vi "mbdmaboot_Host_nodownload.vi"() -> ()   [LabVIEW 2015]
uses:
  <vilib>/FPGAPlugInAG/USRP X310; 294xR; 295xR/niLvFpga_Open_USRP X310; 294xR; 295xR.vi
  <vilib>/rvi/interface/common/dynamic/niFpgaDynamicAddResources.vi
  <vilib>/FPGAPlugInAG/Dynamic/niLvFpga_Download_Dynamic.vi
  <vilib>/FPGAPlugInAG/Dynamic/niLvFpga_Run_Dynamic.vi
  <vilib>/Utility/error.llb/Error Cluster From Error Code.vi
  <vilib>/rvi/errors/niLvFpgaAdjustHostInterfaceError.vi
  <vilib>/FPGAPlugInAG/Dynamic/niLvFpga_Close_Dynamic.vi
  <vilib>/rvi/interface/nirviOpenFPGA/nirviOpenFPGA.xnode
  FPGA Bitfiles/mb-dmaboot_FPGATarget_mbdmaboottopLeve_XKhxGc+VYWY.lvbitx
  <vilib>/rvi/interface/nirviMethod/nirviMethod.xnode
  <vilib>/rvi/interface/nirviReadWriteControl/nirviReadWriteControl.xnode
  <vilib>/rvi/interface/nirviCloseFPGA/nirviCloseFPGA.xnode
  <vilib>/FPGAPlugInAG/Dynamic/niLvFpga_ReadFifo_Dynamic.vi
  <vilib>/rvi/errors/niLvFpgaMergeErrorWithErrorCode.vi
  NiFpgaLv.dll
  <vilib>/rvi/interface/Simulation/niFpgaSimulationCallBeginRW.vi
panel:
  in  "ub1\\reset_rtl":bool
  out "Console out (readonly) 2":string
  out "C":u32
  in  "B":u32
  in  "A":u32
  in  "stop":bool
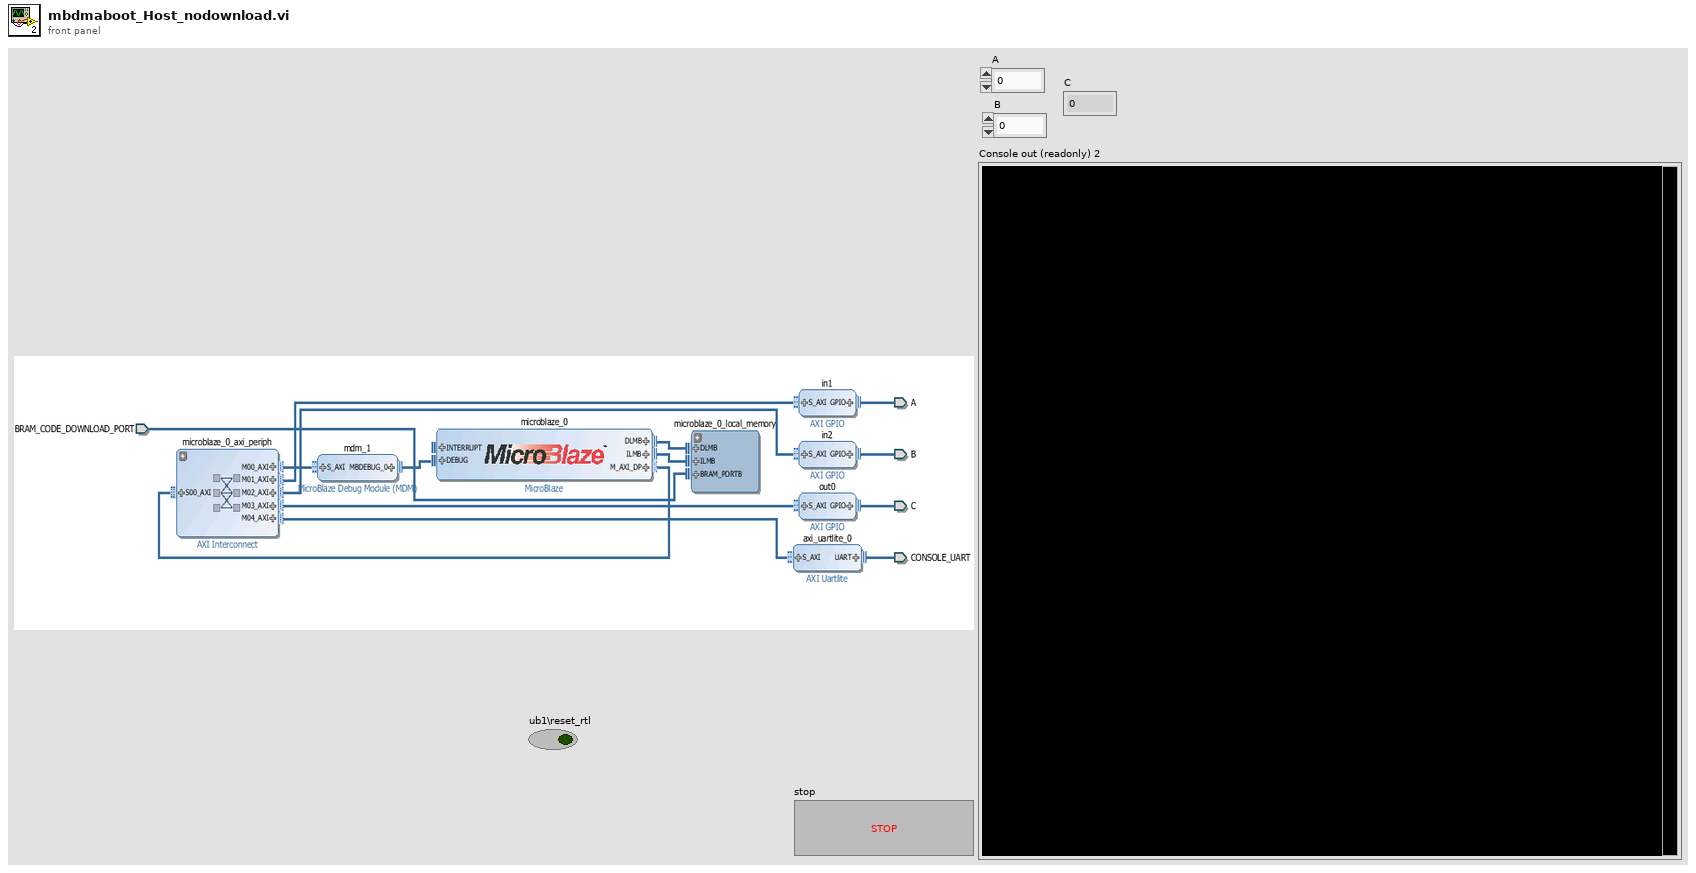
[diagram p1: front panel]
types:
  T1 = cluster{"Baud (ticks)":u32, "CharacterSize":u8, "Parity":enum8{"None", "Even", "Odd"}, "Stop Bits":enum8{"1.0", "1.5", "2.0"}, "Spacing (ticks)":u32}
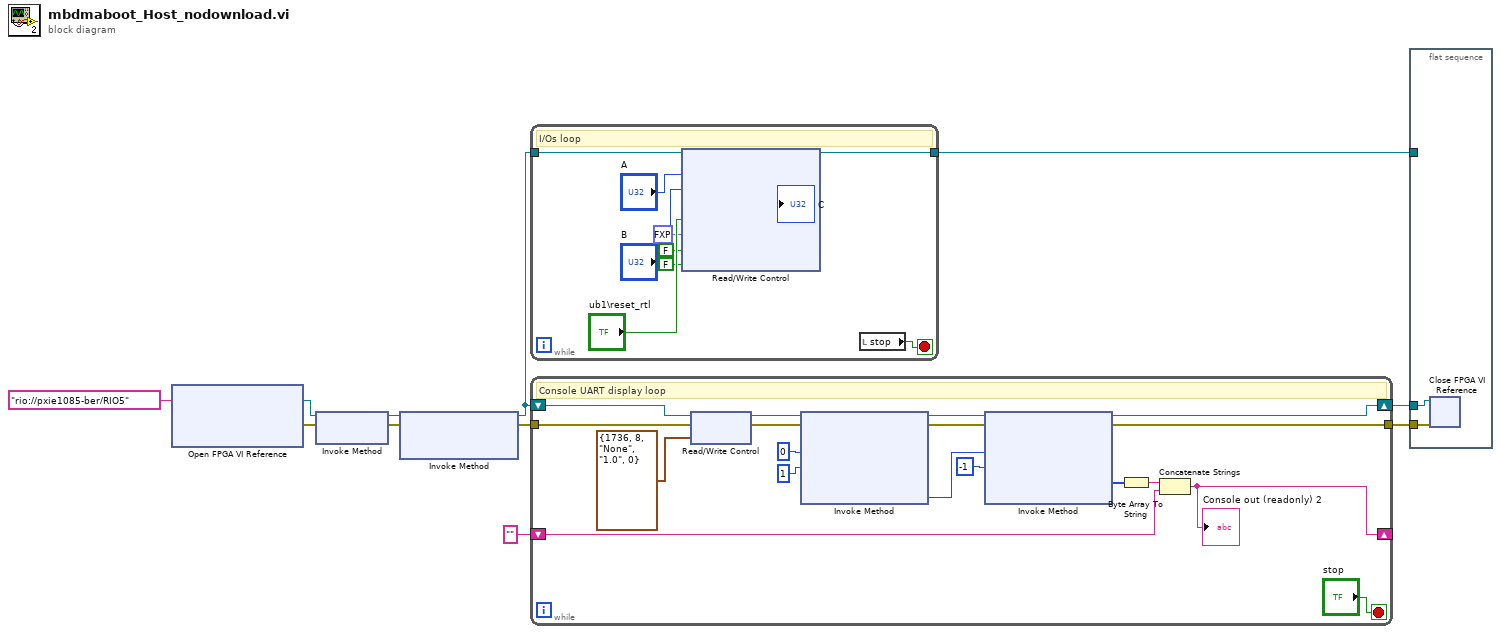
[diagram p0: block diagram]
diagram:
  n1 = xnode "Open FPGA VI Reference"("resource name"=tag "rio://pxie1085-ber/RIO5") -> ("FPGA VI Reference Out"=w11:refnum<k20>, "error out"=w9:errorcluster)  [unwired: 1 in]
  n2 = xnode "Invoke Method"("FPGA VI Reference In"=w11, "error in"=w9) -> ("FPGA VI Reference Out"=w10:refnum<k20>, "error out"=w8:errorcluster)
  n3 = xnode "Invoke Method"("FPGA VI Reference In"=w10, "error in"=w8) -> ("FPGA VI Reference Out"=w2:refnum<k20>, "error out"=w6:errorcluster)  [unwired: 1 in]
  n4 = while {
    tunnel: w2 -> [w21]
    tunnel: [w16] -> w1
    stop <- w17 stop-if-true
    # "I/Os loop"
    n5 = xnode "Read/Write Control"("FPGA VI Reference In"=w21, "A"="A", "B"="B", "ub1\\reset_rtl"="ub1\\reset_rtl", "ub1\\BRAM_PORTB_we"=fxp<+,4,4> 0.0 ("ub1\\BRAM_PORTB_we"), "ub1\\BRAM_PORTB_en"=FALSE ("ub1\\BRAM_PORTB_en"), "ub1\\BRAM_PORTB_rst"=FALSE ("ub1\\BRAM_PORTB_rst")) -> ("FPGA VI Reference Out"=w16:refnum<k20>, "C"=→"C":u32)  [unwired: 1 in, 1 out]
    n6 = local read "stop"() -> (w17:bool)
  }
  n7 = while {
    shift-right: [w32] -> w7
    shift-left: w2 -> [w39]
    tunnel: w6 -> [w28]
    tunnel: [w33] -> w5
    shift-right: [w22] -> _
    shift-left: "" ("string") -> [w24]
    stop <- "stop" stop-if-true
    # "Console UART display loop"
    n8 = xnode "Read/Write Control"("FPGA VI Reference In"=w39, "error in"=w28, "Settings"=T1 {"Baud (ticks)"=1736, "CharacterSize"=8, "Parity"=enum."None", "Stop Bits"=enum."1.0", "Spacing (ticks)"=0}) -> ("FPGA VI Reference Out"=w29:refnum<k20>, "error out"=w27:errorcluster)
    n9 = xnode "Invoke Method"("FPGA VI Reference In"=w29, "error in"=w27, "Number of Elements"=u32 0, "Timeout (ms)"=1) -> ("FPGA VI Reference Out"=w35:refnum<k20>, "error out"=w34:errorcluster, "Elements Remaining"=w31:u32)  [unwired: 1 out]
    n10 = xnode "Invoke Method"("FPGA VI Reference In"=w35, "error in"=w34, "Number of Elements"=w31, "Timeout (ms)"=-1) -> ("FPGA VI Reference Out"=w32:refnum<k20>, "error out"=w33:errorcluster, "Data"=w23:u16[])  [unwired: 1 out]
    n11 = Byte Array To String(unsigned byte array=w23) -> (string=w25:string)
    n12 = Concatenate Strings(w25, w24) -> (w22:string)
    "Console out (readonly) 2" <- w22
  }
  n13 = flat-sequence {
    tunnel: w7 -> [w41]
    tunnel: w5 -> [w40]
    tunnel: w1 -> [_]
    frame #0 {
      n14 = xnode "Close FPGA VI Reference"("FPGA VI Reference In"=w41, "error in"=w40) -> ()  [unwired: 1 out]
    }
  }
